vi "Read(Variant).vi"(6 "prioritize Cache? (F)":bool, 7 "Qualified Name":string, 8 "error in (no error)":errorcluster, 9 "Name (empty: type name)":string, 10 "Type":variant, 11 "ConfigManager in":refnum<class "ConfigManager.lvclass">) -> (0 "error out":errorcluster, 2 "value":variant, 3 "ConfigManager out":refnum<class "ConfigManager.lvclass">)   [LabVIEW 2013, in "CfgManager.lvlib" / "ConfigManager.lvclass"]
uses:
  ConfigManager.lvclass
  ConfigManager.lvclass/ConfigManager.ctl
  Encoding/Encoding.lvclass
  Encryption/Encryption.lvclass
  Serializer/Serializer.lvclass
  Read Serializer.vi
  Read Encoding.vi
  Read Encryption.vi
  Write.vi
  <vilib>/Utility/VariantDataType/GetTypeInfo.vi
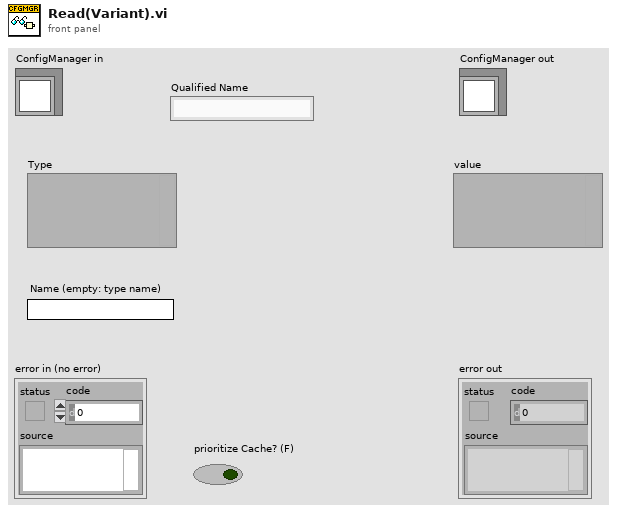
[diagram p1: front panel]
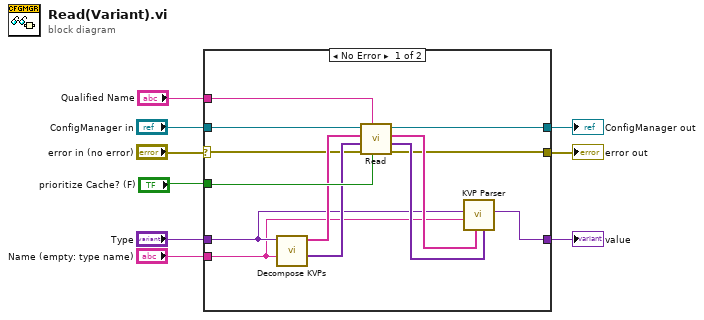
[diagram p0: block diagram]
diagram:
  n1 = case shown="No Error" "error in (no error)" {
    selector: "error in (no error)" -> [w13 w25]
    tunnel: [w12 w25] -> w8
    tunnel: [w11 w24] -> w6
    tunnel: "ConfigManager in" -> [w22 w24]
    tunnel: "Name (empty: type name)" -> [w14 _]
    tunnel: "Type" -> [w15 w23]
    tunnel: [w10 w23] -> w3
    tunnel: "Qualified Name" -> [w21 _]
    tunnel: "prioritize Cache? (F)" -> [w20 _]
    frame No Error {
      n2 = call "Decompose KVPs.vi"("Name (empty: value name)"=w14, "value"=w15) -> ("Values"=w18:variant[], "Keys"=w19:string[])  [unwired: 8 in]
      n3 = call "Read.vi"("prioritize Cache? (F)"=w20, "Qualified Name"=w21, "error in (no error)"=w13, "Default Values"=w18, "keys in"=w19, "ConfigManager in"=w22) -> ("error out"=w12:errorcluster, "Values"=w16:variant[], "keys"=w17:string[], "ConfigManager out"=w11:refnum<class "ConfigManager.lvclass">)  [unwired: 2 in]
      n4 = call <vilib>:"KVP Parser.vi"("Values"=w16, "Keys"=w17, "Default Value Name (empty: label)"=w14, "Default Value"=w15) -> ("Value"=w10:variant)  [unwired: 4 in, 3 out]
    }
    frame Error {
    }
  }
  "error out" <- w8
  "ConfigManager out" <- w6
  "value" <- w3
